vi "Demo - Shortcuts - Pt1.vi"(1 "VISA in":refnum<visa-resource-name>, 3 "error in":errorcluster) -> (7 "error out":errorcluster, 9 "VISA out":refnum<visa-resource-name>)   [LabVIEW 2020]
uses:
  <vilib>/ErrorRing/Error Ring.xnode
panel:
  in  "Stop":bool
  out "LoopNum":i32
  out "Result":dbl
  # "LabVIEW Shortcuts - Pt1"
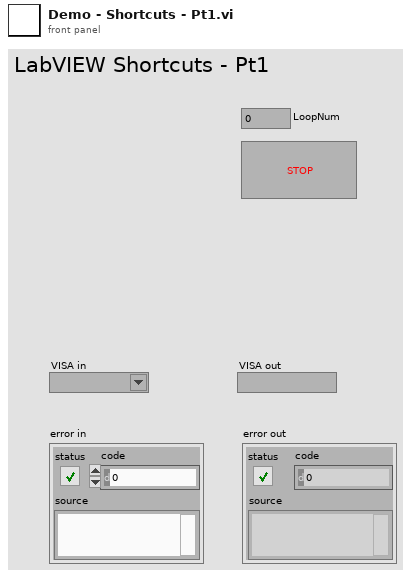
[diagram p1: front panel]
types:
  T1 = enum16{"Wiring - Cleanup Diagram", "Wiring - Change Wire Direction", "Wiring - Wiring Points", "Wiring - Switch Tools", "Wiring - Change Connector Panes", "Execution - Run, Abort and Change Run Edit Mode"}
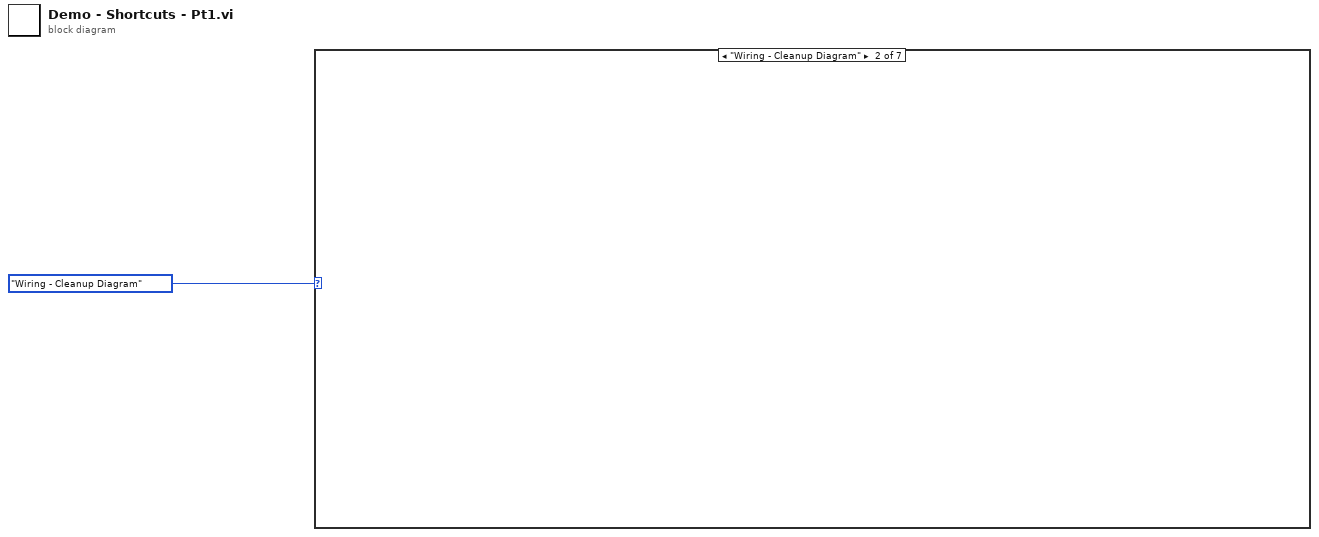
[diagram p0: block diagram]
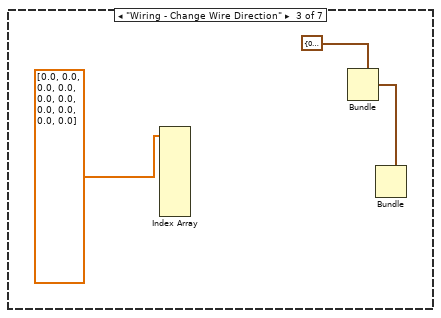
[diagram p3: hidden frame]
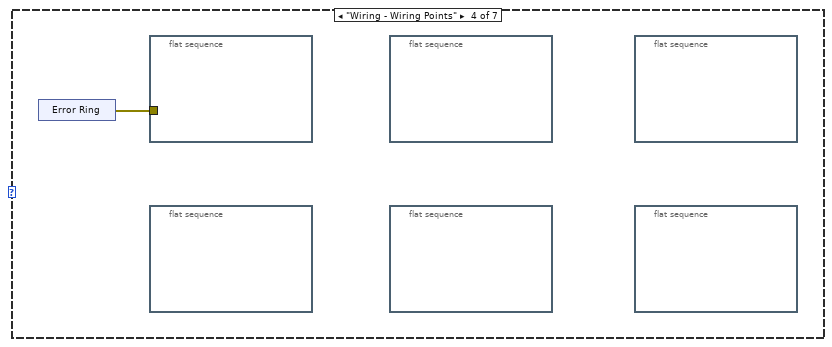
[diagram p4: hidden frame]
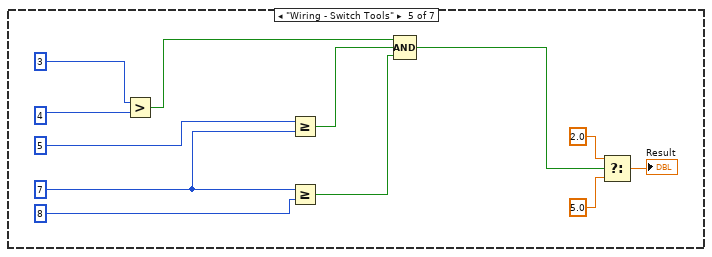
[diagram p5: hidden frame]
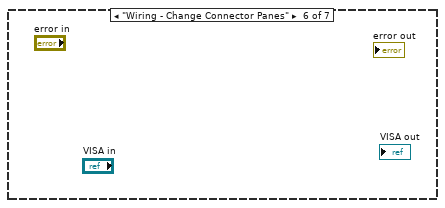
[diagram p6: hidden frame]
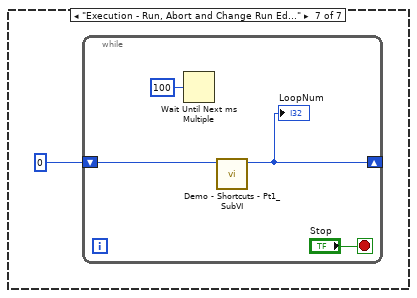
[diagram p7: hidden frame]
diagram:
  n1 = case shown="\"Wiring - Cleanup Diagram\"" T1."Wiring - Cleanup Diagram" {
    frame Default {
      # "Nothing to DEMO"
    }
    frame "Wiring - Cleanup Diagram" {
    }
    frame "Wiring - Change Wire Direction" {
      n2 = Index Array(array=dbl[] [0.0, 0.0, 0.0, 0.0, 0.0, 0.0, 0.0, 0.0, 0.0, 0.0]) -> ()  [unwired: 9 in, 9 out]
      n3 = Bundle(cluster=cluster{dbl, dbl, dbl, dbl} {0.0, 0.0, 0.0, 0.0}) -> (w2:cluster{dbl, dbl, dbl, dbl})  [unwired: 4 in]
      n4 = Bundle(cluster=w2) -> ()  [unwired: 4 in, 1 out]
    }
    frame "Wiring - Wiring Points" {
      n5 = xnode "Error Ring"() -> ("error out"=w5:errorcluster)
      n6 = flat-sequence {
        tunnel: w5 -> [_]
        frame #0 {
        }
      }
      n7 = flat-sequence {
        frame #0 {
        }
      }
      n8 = flat-sequence {
        frame #0 {
        }
      }
      n9 = flat-sequence {
        frame #0 {
        }
      }
      n10 = flat-sequence {
        frame #0 {
        }
      }
      n11 = flat-sequence {
        frame #0 {
        }
      }
    }
    frame "Wiring - Switch Tools" {
      w12 = 7
      n12 = Greater?(x=3, y=4) -> (0:w15:bool)
      n13 = Greater Or Equal?(x=5, y=w12) -> (x >= y?=w14:bool)
      n14 = Greater Or Equal?(x=w12, y=8) -> (x >= y?=w7:bool)
      n15 = Compound Arithmetic op=AND(w15, w14, w7) -> (w13:bool)
      n16 = Select(t=2.0, s=w13, f=5.0) -> (s? t:f=→"Result":dbl)
    }
    frame "Wiring - Change Connector Panes" {
    }
    frame "Execution - Run, Abort and Change Run Edit Mode" {
      n17 = while {
        shift-right: [w21] -> _
        shift-left: 0 -> [w22]
        stop <- "Stop" stop-if-true
        n18 = Wait Until Next ms Multiple(millisecond multiple=u32 100) -> ()  [unwired: 1 out]
        n19 = call "Demo - Shortcuts - Pt1_ SubVI.vi"("NumIn"=w22) -> ("NumOut"=w21:i32)  [unwired: 10 in]
        "LoopNum" <- w21
      }
    }
  }
